vi "Configure Measurement.vi"   [LabVIEW 2017, in "Agilent 6000 Series.lvlib"]
doc: "This VI configures the measurement."
uses:
  <instrlib>/Agilent 6000 Series/Agilent 6000 Series.lvlib
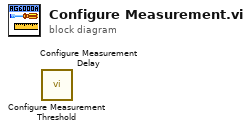
[diagram p0: block diagram]
diagram:
  n1 = call <instrlib>:"Configure Measurement Threshold.vi"() -> ()  [unwired: 10 in, 2 out]
  n2 = call <instrlib>:"Configure Measurement Delay.vi"() -> ()  [unwired: 10 in, 2 out]
